vi "Rotational.vi"(3 "Joy Z":dbl) -> (1 "Omega":dbl)   [LabVIEW 2014]
uses:
  <vilib>/Rock Robotics/Network Tables/SD Write Number.vi
  Robot Global Data.vi
  <vilib>/addons/control/pid/pid.llb/PID (DBL).vi
  <vilib>/addons/control/pid/NI_PID_pid.lvlib
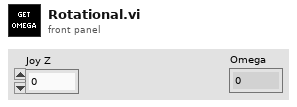
[diagram p1: front panel]
types:
  T1 = typedef "WPI_GyroDevRef.ctl" = cluster{"DevStatus":errorcluster, "Analog Module":T2, "Analog Channel":T3, "Offset":dbl, "Gain (VoltsPerDegree/Second)":dbl}
  T2 = typedef "FPGA_TypedefAnalogModule.ctl" = enum16{"Controller 1"}
  T3 = typedef "FPGA_AIChannel.ctl" = enum8{"AI 0", "AI 1", "AI 2", "AI 3", "AI MXP 0", "AI MXP 1", "AI MXP 2", "AI MXP 3", "Invalid"}
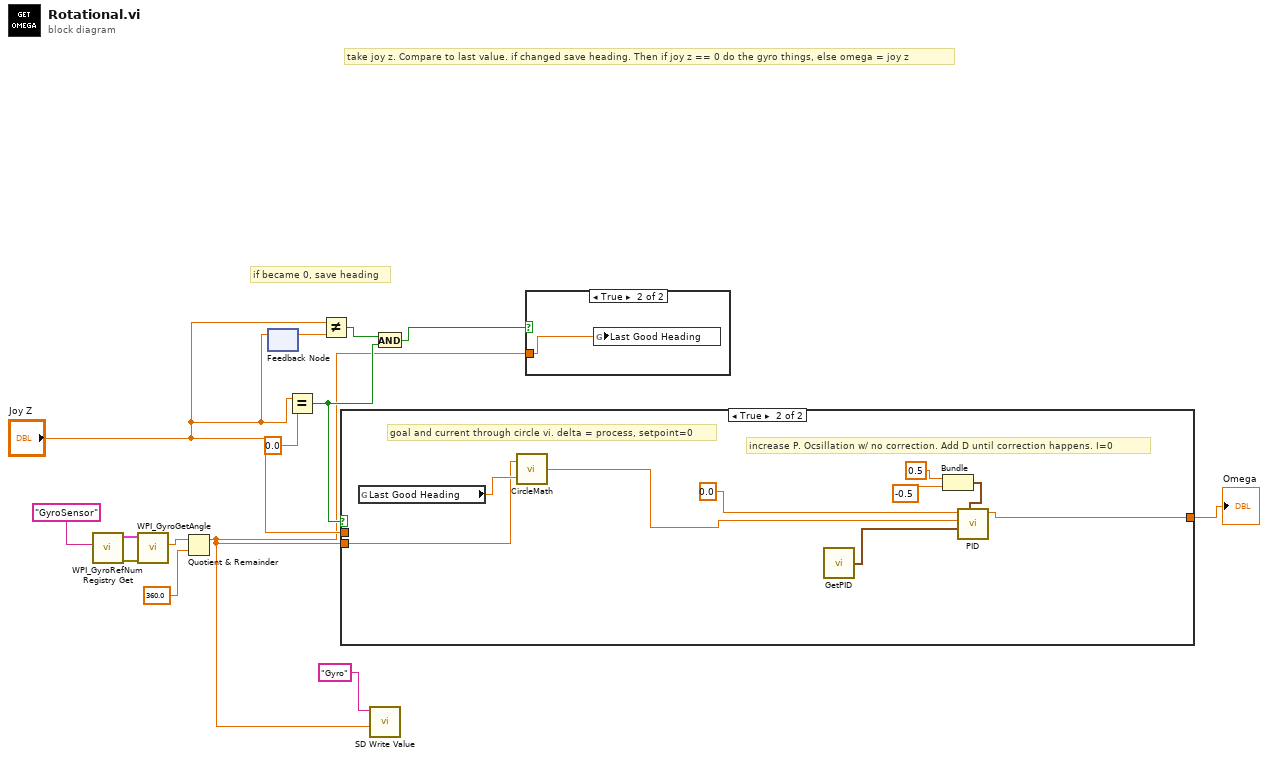
[diagram p0: block diagram]
diagram:
  # "take joy z. Compare to last value. if changed save heading. Then if joy z == 0 do the gyro things, else omega = joy z"
  # "if became 0, save heading"
  n1 = call <vilib>:"WPI_GyroRefNum Registry Get.vi"("refnum name"="GyroSensor") -> ("error out"=w14:errorcluster, "GyroDevRef"=w13:T1)  [unwired: 9 in]
  n2 = call <vilib>:"WPI_GyroGetAngle.vi"("error in (no error)"=w14, "GyroDevRef"=w13) -> ("Angle"=w4:dbl)  [unwired: 6 in, 3 out]
  n3 = Quotient & Remainder(x=w4, y=360.0) -> (x-y*floor(x/y)=w1:dbl)  [unwired: 1 out]
  n4 = feedback #1() -> (w11:dbl)  [unwired: 1 in]
  n5 = feedback-in #1("Joy Z") -> ()
  n6 = Equal?(x="Joy Z", y=0.0) -> (x = y?=w7:bool)
  n7 = Not Equal?(x="Joy Z", y=w11) -> (x != y?=w9:bool)
  n8 = case shown="True" w7 {
    tunnel: [w15 w18] -> w6
    tunnel: w1 -> [_ w17]
    tunnel: "Joy Z" -> [w15 _]
    frame False {
    }
    frame True {
      # "goal and current through circle vi. delta = process, setpoint=0"
      # "increase P. Ocsillation w/ no correction. Add D until correction happens. I=0"
      n9 = global read "Robot Global Data.vi" "Last Good Heading"() -> (w20:dbl)
      n10 = call "CircleMath.vi"("Target Heading"=w20, "Current Heading"=w17) -> ("Delta Heading"=w19:dbl)
      n11 = call "GetPID.vi"() -> ("PID Gains"=w16:cluster{"P":dbl, "I":dbl, "D":dbl})
      n12 = Bundle(0.5, -0.5) -> (w22:cluster{dbl, dbl})  [unwired: 1 in]
      n13 = call-poly <vilib>:"PID.vi"("output range"=w22, "PID gains"=w16, "process variable"=w19, "setpoint"=0.0) -> ("output"=w18:dbl)  [unwired: 6 in, 1 out]
    }
  }
  "Omega" <- w6
  n14 = call-poly <vilib>:"SD Write Value.vi"("Numeric"=w1, "Name"="Gyro") -> ()  [unwired: 8 in, 2 out]
  n15 = And(x=w9, y=w7) -> (x .and. y?=w8:bool)
  n16 = case shown="True" w8 {
    tunnel: w1 -> [_ w25]
    frame False {
    }
    frame True {
      n17 = global write "Robot Global Data.vi" "Last Good Heading"(w25) -> ()
    }
  }
